vi "Host - Find Path.vi"(7 "Type":enum16{"Slave", "Master"}(ring), 8 "error in (no error)":errorcluster, 9 "Slave Index":u32, 10 "Master Index":u32, 11 "serverName":string="10.0.18.167") -> (0 "error out":errorcluster, 2 "Path":string)   [LabVIEW 2016, in "Scan Engine Custom Device.lvlib"]
uses:
  Scan Engine Custom Device.lvlib
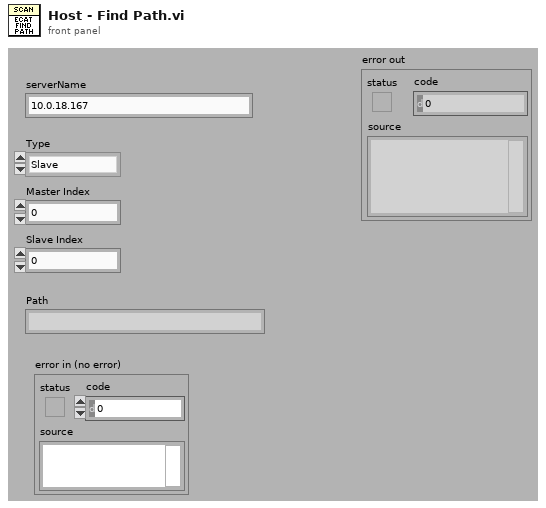
[diagram p1: front panel]
types:
  T1 = typedef "Scan Engine Custom Device.lvlib/Host - HW Config.ctl" = cluster{"Local Chassis":T2, "Masters":T4[]}
  T2 = typedef "Scan Engine Custom Device.lvlib/Host - Local Chassis.ctl" = cluster{"Modules":T3[]}
  T3 = typedef "Scan Engine Custom Device.lvlib/Host - Module.ctl" = cluster{"IOV Ref":refnum<k21>, "Slot":u32, "Model":u32}
  T4 = typedef "Scan Engine Custom Device.lvlib/Host - Master.ctl" = cluster{"IOV Ref":refnum<k21>, "Name":string, "Master ID":u32, "Slaves":T5[]}
  T5 = typedef "Scan Engine Custom Device.lvlib/Host - Slave.ctl" = cluster{"IOV Ref":refnum<k21>, "Name":string, "Position Address":u16, "Bitfile Signature":u8[], "Modules":T3[], "ECAT Variablenobjekt":refnum<k21>[]}
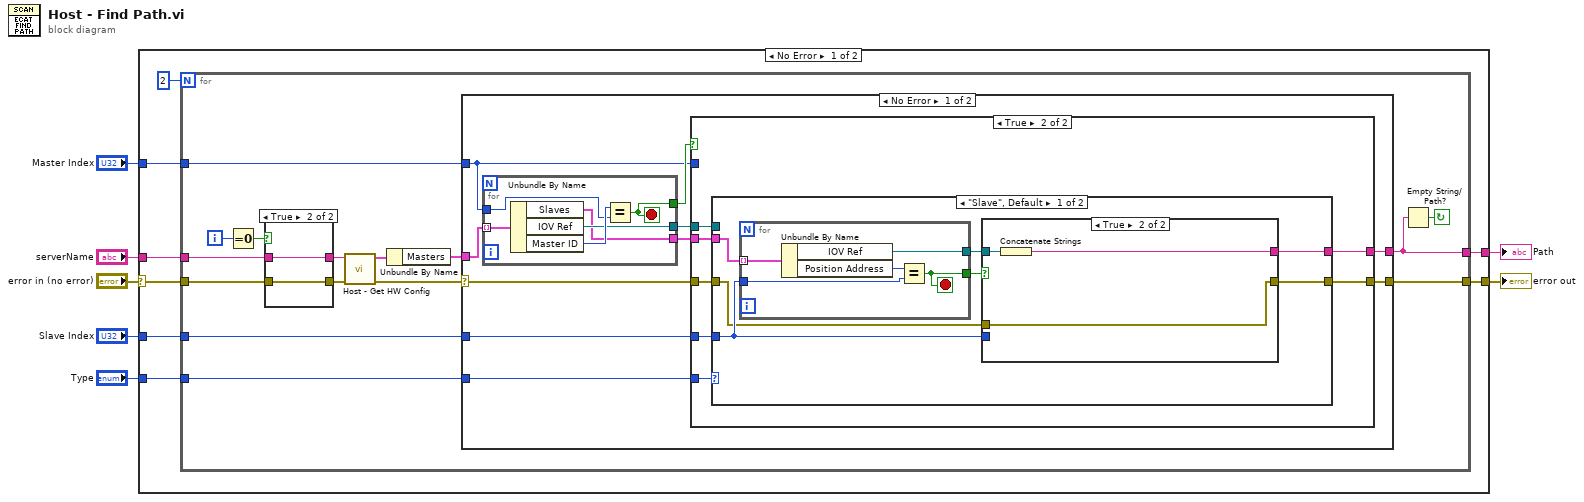
[diagram p0: block diagram]
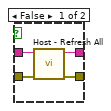
[diagram p2: hidden frame]
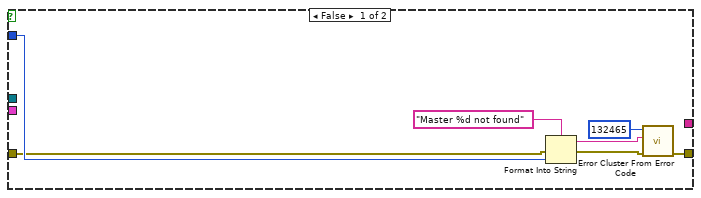
[diagram p3: hidden frame]
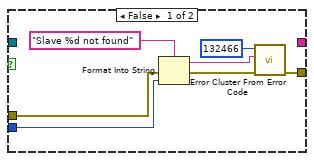
[diagram p4: hidden frame]
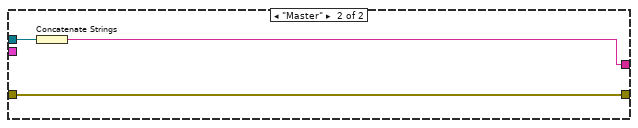
[diagram p5: hidden frame]
diagram:
  n1 = case shown="No Error" "error in (no error)" {
    selector: "error in (no error)" -> [w8 w93]
    tunnel: "Slave Index" -> [w15 _]
    tunnel: "Type" -> [w14 _]
    tunnel: "Master Index" -> [w13 _]
    tunnel: "serverName" -> [w12 _]
    tunnel: [w11 _] -> w3
    tunnel: [w10 w93] -> w2
    frame No Error {
      n2 = for {
        N: 2 -> [_]
        tunnel: w15 -> [w30]
        tunnel: w14 -> [w29]
        tunnel: w13 -> [w28]
        tunnel: w8 -> [w27]
        tunnel: w12 -> [w26]
        tunnel: [w16] -> w11
        tunnel: [w20] -> w10
        i -> [w19]
        stop <- w17 continue-if-true
        n3 = Equal To 0?(x=w19) -> (x = 0?=w18:bool)
        n4 = case shown="True" w18 {
          tunnel: w27 -> [w34 w35]
          tunnel: w26 -> [w33 w36]
          tunnel: [w32 w36] -> w25
          tunnel: [w31 w35] -> w24
          frame False {
            n5 = call "Host - Refresh All.vi"("error in (no error)"=w34, "serverName"=w33) -> ("error out"=w31:errorcluster, "serverName"=w32:string)  [unwired: 8 in]
          }
          frame True {
          }
        }
        n6 = call "Host - Get HW Config.vi"("error in (no error)"=w24, "serverName"=w25) -> ("error out"=w23:errorcluster, "HW Config"=w22:T1)  [unwired: 8 in]
        n7 = Unbundle By Name(w22) -> ("Masters"=w21:T4[])
        n8 = case shown="No Error" w23 {
          selector: w23 -> [w38 w92]
          tunnel: w21 -> [w43 _]
          tunnel: w28 -> [w42 _]
          tunnel: w30 -> [w41 _]
          tunnel: w29 -> [w40 _]
          tunnel: [w39 _] -> w16
          tunnel: [w37 w92] -> w20
          frame No Error {
            n9 = for {
              tunnel: [w91] -> w44
              tunnel: w43 -> [w90] mode=indexing
              tunnel: w42 -> [w88]
              tunnel: [w87] -> w45
              tunnel: [w86] -> w46
              stop <- w91 stop-if-true
              n10 = Unbundle By Name(w90) -> ("Slaves"=w86:T5[], "IOV Ref"=w87:refnum<k21>, "Master ID"=w89:u32)
              n11 = Equal?(x=w89, y=w88) -> (x = y?=w91:bool)
            }
            n12 = case shown="True" w44 {
              tunnel: w45 -> [_ w59]
              tunnel: w40 -> [_ w60]
              tunnel: [_ w58] -> w39
              tunnel: w41 -> [_ w57]
              tunnel: w46 -> [_ w56]
              tunnel: w42 -> [w49 _]
              tunnel: w38 -> [w48 w54]
              tunnel: [w47 w55] -> w37
              frame False {
                n13 = Format Into String(format string="Master %d not found", error in=w48, w49) -> (resulting string=w51:string, error out=w50:errorcluster)  [unwired: 1 in]
                n14 = call <vilib>:"Error Cluster From Error Code.vi"("error in (no error)"=w50, "error message (\"\")"=w51, "error code (0)"=132465) -> ("error out"=w47:errorcluster)  [unwired: 6 in]
              }
              frame True {
                n15 = case shown="\"Slave\", Default" w60 {
                  tunnel: w59 -> [_ w84]
                  tunnel: [w66 w83] -> w58
                  tunnel: w57 -> [w65 _]
                  tunnel: w56 -> [w64 _]
                  tunnel: [w61 w85] -> w55
                  tunnel: w54 -> [w62 w85]
                  frame "Slave", Default {
                    n16 = for {
                      tunnel: w65 -> [w82]
                      tunnel: [w81] -> w67
                      tunnel: w64 -> [w80] mode=indexing
                      tunnel: [w78] -> w63
                      stop <- w81 stop-if-true
                      n17 = Unbundle By Name(w80) -> ("IOV Ref"=w78:refnum<k21>, "Position Address"=w79:u16)
                      n18 = Equal?(x=w79, y=w82) -> (x = y?=w81:bool)
                    }
                    n19 = case shown="True" w67 {
                      tunnel: [_ w75] -> w66
                      tunnel: w65 -> [w70 _]
                      tunnel: w63 -> [_ w76]
                      tunnel: w62 -> [w69 w77]
                      tunnel: [w68 w77] -> w61
                      frame False {
                        n20 = Format Into String(format string="Slave %d not found", error in=w69, w70) -> (resulting string=w72:string, error out=w71:errorcluster)  [unwired: 1 in]
                        n21 = call <vilib>:"Error Cluster From Error Code.vi"("error in (no error)"=w71, "error message (\"\")"=w72, "error code (0)"=132466) -> ("error out"=w68:errorcluster)  [unwired: 6 in]
                      }
                      frame True {
                        n22 = Concatenate Strings(w76) -> (w75:string)
                      }
                    }
                  }
                  frame "Master" {
                    n23 = Concatenate Strings(w84) -> (w83:string)
                  }
                }
              }
            }
          }
          frame Error {
          }
        }
        n24 = Empty String/Path?(string/path=w16) -> (empty?=w17:bool)
      }
    }
    frame Error {
    }
  }
  "error out" <- w2
  "Path" <- w3
